vi "CryoServer Test Program.vi"(8 "error in (no error)":errorcluster) -> (0 "error out":errorcluster)   [LabVIEW 2019]
uses:
  CryoServer.lvclass
panel:
  in  "address":string
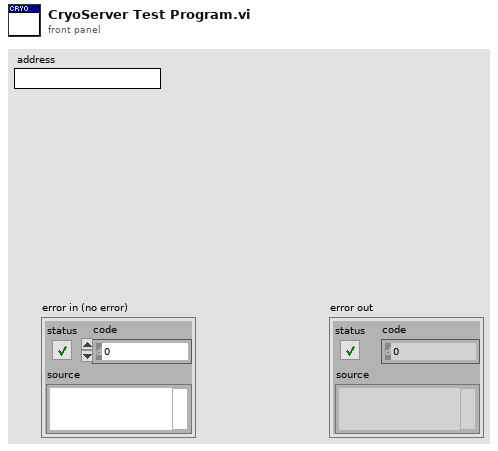
[diagram p1: front panel]
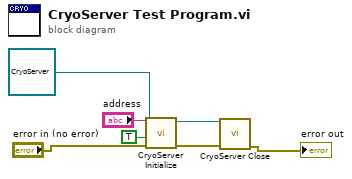
[diagram p0: block diagram]
diagram:
  n1 = call-dynamic "CryoServer Initialize.vi"("error in (no error)"="error in (no error)", "Show GUI? (False)"=TRUE, "address"="address", "CryoServer in"=refnum<class "CryoServer.lvclass"> refnum) -> ("error out"=w4:errorcluster, "CryoServer out"=w5:refnum<class "CryoServer.lvclass">)  [unwired: 6 in]
  n2 = call-dynamic "CryoServer Close.vi"("error in (no error)"=w4, "CryoServer in"=w5) -> ("error out"=→"error out":errorcluster)  [unwired: 8 in, 1 out]
